vi "Main - Fan Module Test Program[Student].vi"() -> ()   [LabVIEW 2017]
panel:
  in  "DAQmx Device Name":tag="myDAQ1"
  in  "Zero Power":bool
  in  "Full Power":bool
  in  "Clear Graph":bool
  out "Fan Output":dbl(graph)
  in  "stop":bool
  in  "Fan Power":dbl(slide) scale=0.0..10.0
  out "Loop Time":u32
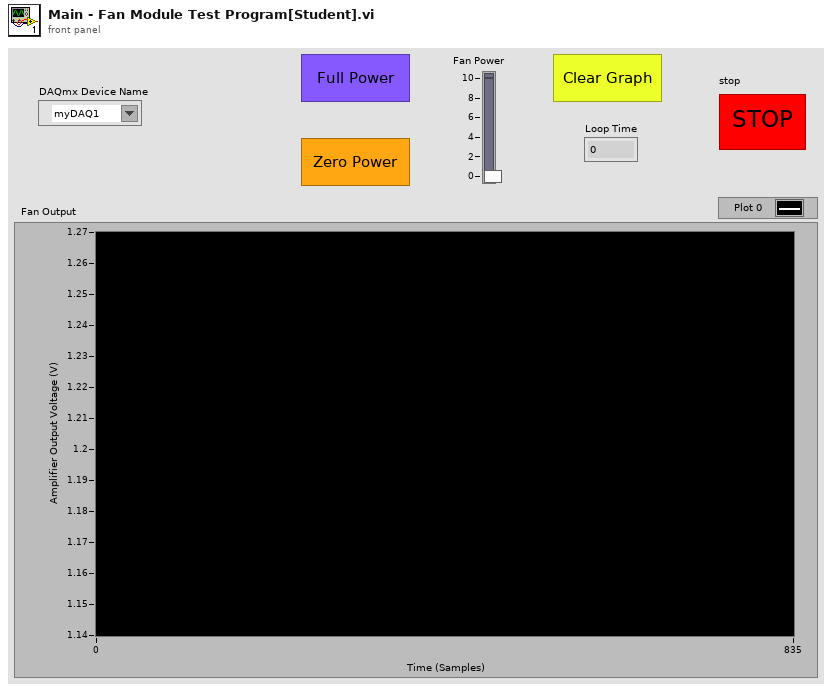
[diagram p1: front panel]
types:
  T1 = cluster{"AI Task":refnum<k21>, "Ctr0 Task":refnum<k21>, "Ao Task":refnum<k21>, "DO Task":refnum<k21>}
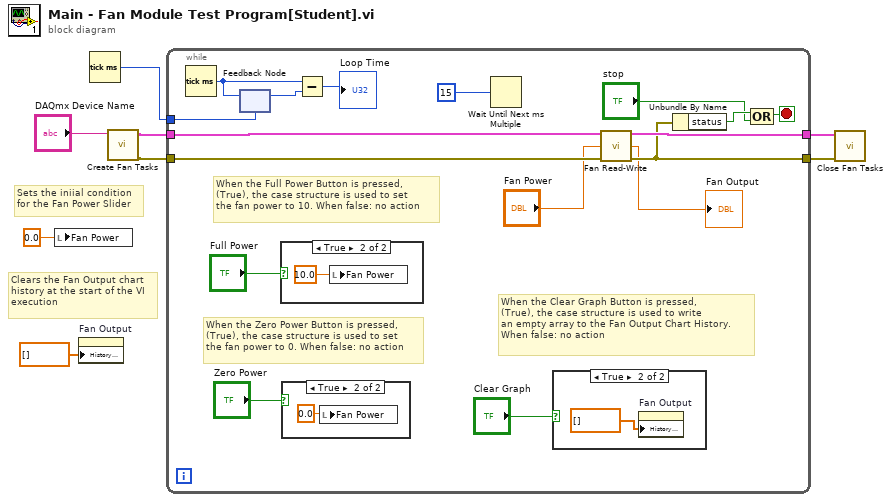
[diagram p0: block diagram]
diagram:
  # "Clears the Fan Output chart\nhistory at the start of the VI\nexecution"
  # "Sets the iniial condition\nfor the Fan Power Slider"
  n1 = local write "Fan Power"(0.0 ("Slide")) -> ()
  n2 = property on="Fan Output" class="WFChart (strict)"("History Data"=dbl[] []) -> ()  [unwired: 2 in, 2 out]
  n3 = Tick Count (ms)() -> (millisecond timer value=w3:u32)
  n4 = call "Create Fan Tasks.vi"("DAQmx Device Name"="DAQmx Device Name") -> ("Error Out"=w7:errorcluster, "Hellicopter Tasks Output"=w8:T1)  [unwired: 5 in]
  n5 = while {
    tunnel: w7 -> [w22]
    tunnel: w8 -> [w23]
    tunnel: [w21] -> w5
    tunnel: [w20] -> w6
    tunnel: w3 -> [w19]
    stop <- w25 stop-if-true
    # "When the Clear Graph Button is pressed,\n(True), the case structure is used to write\nan empty array to the Fan Output Chart History.\nWhen false: no action"
    # "When the Zero Power Button is pressed,\n(True), the case structure is used to set\nthe fan power to 0. When false: no action"
    # "When the Full Power Button is pressed,\n(True), the case structure is used to set\nthe fan power to 10. When false: no action"
    n6 = Tick Count (ms)() -> (millisecond timer value=w17:u32)
    n7 = feedback-in #1(w17) -> ()
    n8 = feedback #1(w19) -> (w18:u32)
    n9 = case shown="True" "Full Power" {
      frame False {
      }
      frame True {
        n10 = local write "Fan Power"(10.0 ("Slide")) -> ()
      }
    }
    n11 = case shown="True" "Zero Power" {
      frame False {
      }
      frame True {
        n12 = local write "Fan Power"(0.0 ("Slide")) -> ()
      }
    }
    n13 = Subtract(x=w17, y=w18) -> (x-y=→"Loop Time":u32)
    n14 = Wait Until Next ms Multiple(millisecond multiple=u32 15) -> ()  [unwired: 1 out]
    n15 = case shown="True" "Clear Graph" {
      frame False {
      }
      frame True {
        n16 = property on="Fan Output" class="WFChart (strict)"("History Data"=dbl[] []) -> ()  [unwired: 2 in, 2 out]
      }
    }
    n17 = call "Fan Read-Write.vi"("Hellicopter Tasks Input"=w23, "Fan Input"="Fan Power", "Error In"=w22) -> ("Hellicopter Tasks Output"=w21:T1, "L/C Output"=→"Fan Output":dbl, "Error Out"=w20:errorcluster)  [unwired: 10 in]
    n18 = Unbundle By Name(w20) -> ("status"=w24:bool)
    n19 = Compound Arithmetic op=OR(w24, "stop") -> (w25:bool)
  }
  n20 = call "Close Fan Tasks.vi"("Error In"=w6, "Hellicopter Tasks Input 2"=w5) -> ()  [unwired: 9 in, 1 out]
